vi "Comm_close 1d dbl waveform.vi"(8 "error in (no error)":errorcluster, 11 "WPL Comm (1D DBL) in":refnum<class "WPL Comm (1D DBL).lvclass">) -> (0 "error out":errorcluster)   [LabVIEW 2020, in "Internal Comm Classes.lvlib" / "WPL Comm (1D DBL).lvclass"]
uses:
  WPL Comm (1D DBL).lvclass
  D:/p4/penguin/lvaddon/Veristand/master/src/LabVIEW/vilib/NI VeriStand/Custom Device Waveform API/Internal Comm Classes/WPL Comm/WPL Comm.lvclass
  WPL Comm.lvclass/WPL Comm.ctl
  WPL Comm (1D DBL).lvclass/WPL Comm (1D DBL).ctl
  WPL Command.ctl
  Set ErrorQ on Variant.vi
  Send WPL Command.vi
  WPL Comm.lvclass
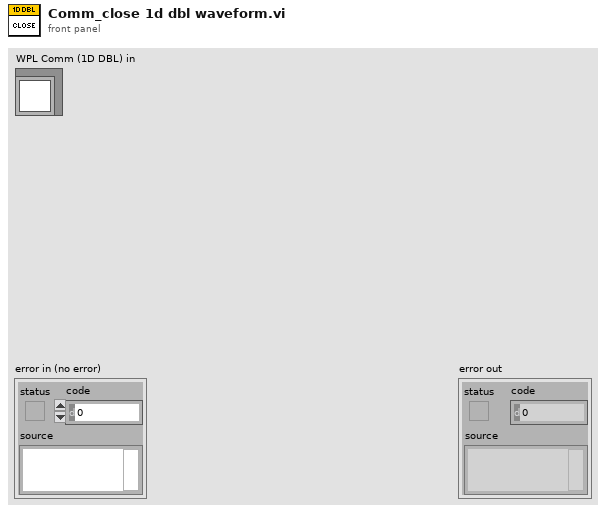
[diagram p1: front panel]
types:
  T1 = typedef "NI_VS Custom Device Waveform API.lvlib/Access mode.ctl" = enum16{"Read", "Write"}
  T2 = typedef "Internal Comm Classes.lvlib/WPL Comm.lvclass/WPL Command.ctl" = enum16{"Register 1D DBL Reader", "Unregister 1D DBL Reader", "Register 1D DBL Writer", "Register 2D DBL Writer", "Unregister 1D DBL Writer", "Unregister 2D DBL Writer", "DBL WFM Start", "WFM 1D DBL Data", "WFM 2D DBL Data", "Shut down", "Handle Error", "Register 1D CDB Reader", "Unregister 1D CDB Reader", "Register 1D CDB Writer", "Unregister 1D CDB Writer", "Register 2D CDB Writer", "Unregister 2D CDB Writer", "WFM 1D CDB Data", "WFM 2D CDB Data", "CDB WFM Start", "Error Shutdown", "Register Streams", "Unregister Streams", "Delete All Streams", "Get WFM DTs", "DBL WFM Multi Start", "CDB WFM Multi Start"}
  T3 = typedef "Internal Comm Classes.lvlib/WPL Comm (1D DBL).lvclass/Waveform 1d dbl read queue.ctl" = refnum<queue>
  T4 = typedef "Internal Comm Classes.lvlib/WPL Comm (1D DBL).lvclass/Waveform 1d dbl queue.ctl" = refnum<queue>
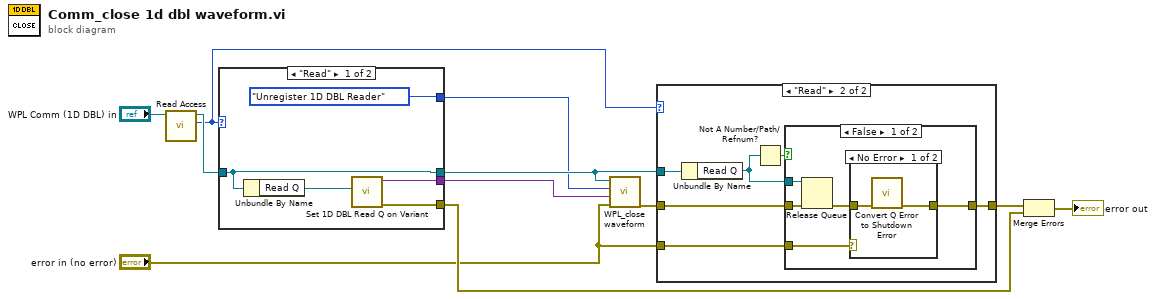
[diagram p0: block diagram]
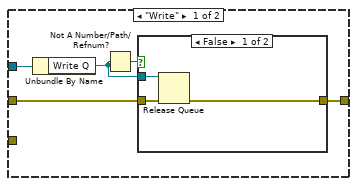
[diagram p2: hidden frame]
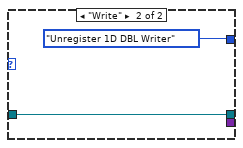
[diagram p6: hidden frame]
diagram:
  n1 = call "Read Access.vi"("WPL Comm in"="WPL Comm (1D DBL) in") -> ("Access"=w4:T1, "WPL Comm out"=w7:refnum<class "WPL Comm (1D DBL).lvclass">)  [unwired: 9 in]
  n2 = case shown="\"Read\"" w4 {
    tunnel: [WPL_Command."Unregister 1D DBL Reader" ("Command") WPL_Command."Unregister 1D DBL Writer" ("Command")] -> w3
    tunnel: w7 -> [w14 w17]
    tunnel: [w14 w17] -> w5
    tunnel: [w15 _] -> w6
    tunnel: [w12 _] -> w2
    frame "Read" {
      n3 = Unbundle By Name(w14) -> ("Read Q"=w13:T3)
      n4 = call "Set 1D DBL Read Q on Variant.vi"("1D DBL Read Q"=w13) -> ("error out"=w15:errorcluster, "Variant out"=w12:variant)  [unwired: 8 in, 1 out]
    }
    frame "Write" {
    }
  }
  n5 = call "WPL_close waveform.vi"("error in (no error)"="error in (no error)", "Variant"=w2, "Command"=w3, "WPL Comm in"=w5) -> ("error out"=w9:errorcluster)  [unwired: 7 in]
  n6 = case shown="\"Read\"" w4 {
    tunnel: w9 -> [w23 w33]
    tunnel: [w22 w32] -> w8
    tunnel: w5 -> [w21 w31]
    tunnel: "error in (no error)" -> [_ w28]
    frame "Write" {
      n7 = Unbundle By Name(w21) -> ("Write Q"=w20:T4)
      n8 = Not A Number/Path/Refnum?(number/path/refnum=w20) -> (NaN/Path/Refnum?=w19:bool)
      n9 = case shown="False" w19 {
        tunnel: w23 -> [w26 w27]
        tunnel: [w25 w27] -> w22
        tunnel: w20 -> [w24 _]
        frame False {
          n10 = Release Queue(queue=w24, error in (no error)=w26) -> (error out=w25:errorcluster)  [unwired: 1 in, 2 out]
        }
        frame True {
        }
      }
    }
    frame "Read" {
      n11 = Unbundle By Name(w31) -> ("Read Q"=w30:T3)
      n12 = Not A Number/Path/Refnum?(number/path/refnum=w30) -> (NaN/Path/Refnum?=w29:bool)
      n13 = case shown="False" w29 {
        tunnel: w33 -> [w38 w42]
        tunnel: [w35 w42] -> w32
        tunnel: w30 -> [w37 _]
        tunnel: w28 -> [w34 _]
        frame False {
          n14 = Release Queue(queue=w37, error in (no error)=w38) -> (error out=w36:errorcluster)  [unwired: 1 in, 2 out]
          n15 = case shown="No Error" w34 {
            tunnel: w36 -> [w40 w41]
            tunnel: [w39 w41] -> w35
            frame No Error {
              n16 = call "Convert Q Error to Shutdown Error.vi"("error in (no error)"=w40) -> ("error out"=w39:errorcluster)  [unwired: 10 in]
            }
            frame Error {
            }
          }
        }
        frame True {
        }
      }
    }
  }
  n17 = Merge Errors(w8, w6) -> (→"error out":errorcluster)
